vi "SwerveDriveRegisterEachMotor.vi"(8 "error in (no error)":errorcluster, 10 "SwerveDrive refnum name":string="My SwerveDrive RefNum", 11 "SwerveDriveDevRef":T1={"DevStatus"={"status"=FALSE, "code"=0, "source"=""}, "TurnMotors[]"=[], "Square Inputs"=FALSE, "Max Output"=1.0, "DriveMotors[]"=[], "WheelOffset[]"=[], "SwerveSensors[]"=[], "RobotSize"={"Width"=[], "Length"=[], "Center"=[]}}) -> (0 "error out":errorcluster, 3 "SwerveDriveDevRef":T1={"DevStatus"={"status"=FALSE, "code"=0, "source"=""}, "TurnMotors[]"=[], "Square Inputs"=FALSE, "Max Output"=1.0, "DriveMotors[]"=[], "WheelOffset[]"=[], "SwerveSensors[]"=[], "RobotSize"={"Width"=[], "Length"=[], "Center"=[]}})   [LabVIEW 2019, in "Swerve Drive.lvlib"]
doc: "Register each of the motors belonging to RobotDrive."
uses:
  Swerve Drive.lvlib
  SwerveDriveDevRef.ctl
  <vilib>/Rock Robotics/WPI/MotorControl/WPI_MotorControlDeviceRef.ctl
  <vilib>/Rock Robotics/WPI/MotorControl/WPI_MotorControlType.ctl
  <vilib>/Rock Robotics/SystemInterfaces/DIO/FPGA_DIOPWMChannel.ctl
  <vilib>/Rock Robotics/WPI/PWM/WPI_PWMDeadband.ctl
  <vilib>/Rock Robotics/SystemInterfaces/DIO/FPGA_DIOChannel.ctl
  <vilib>/Rock Robotics/SystemInterfaces/AI/FPGA_AIChannel.ctl
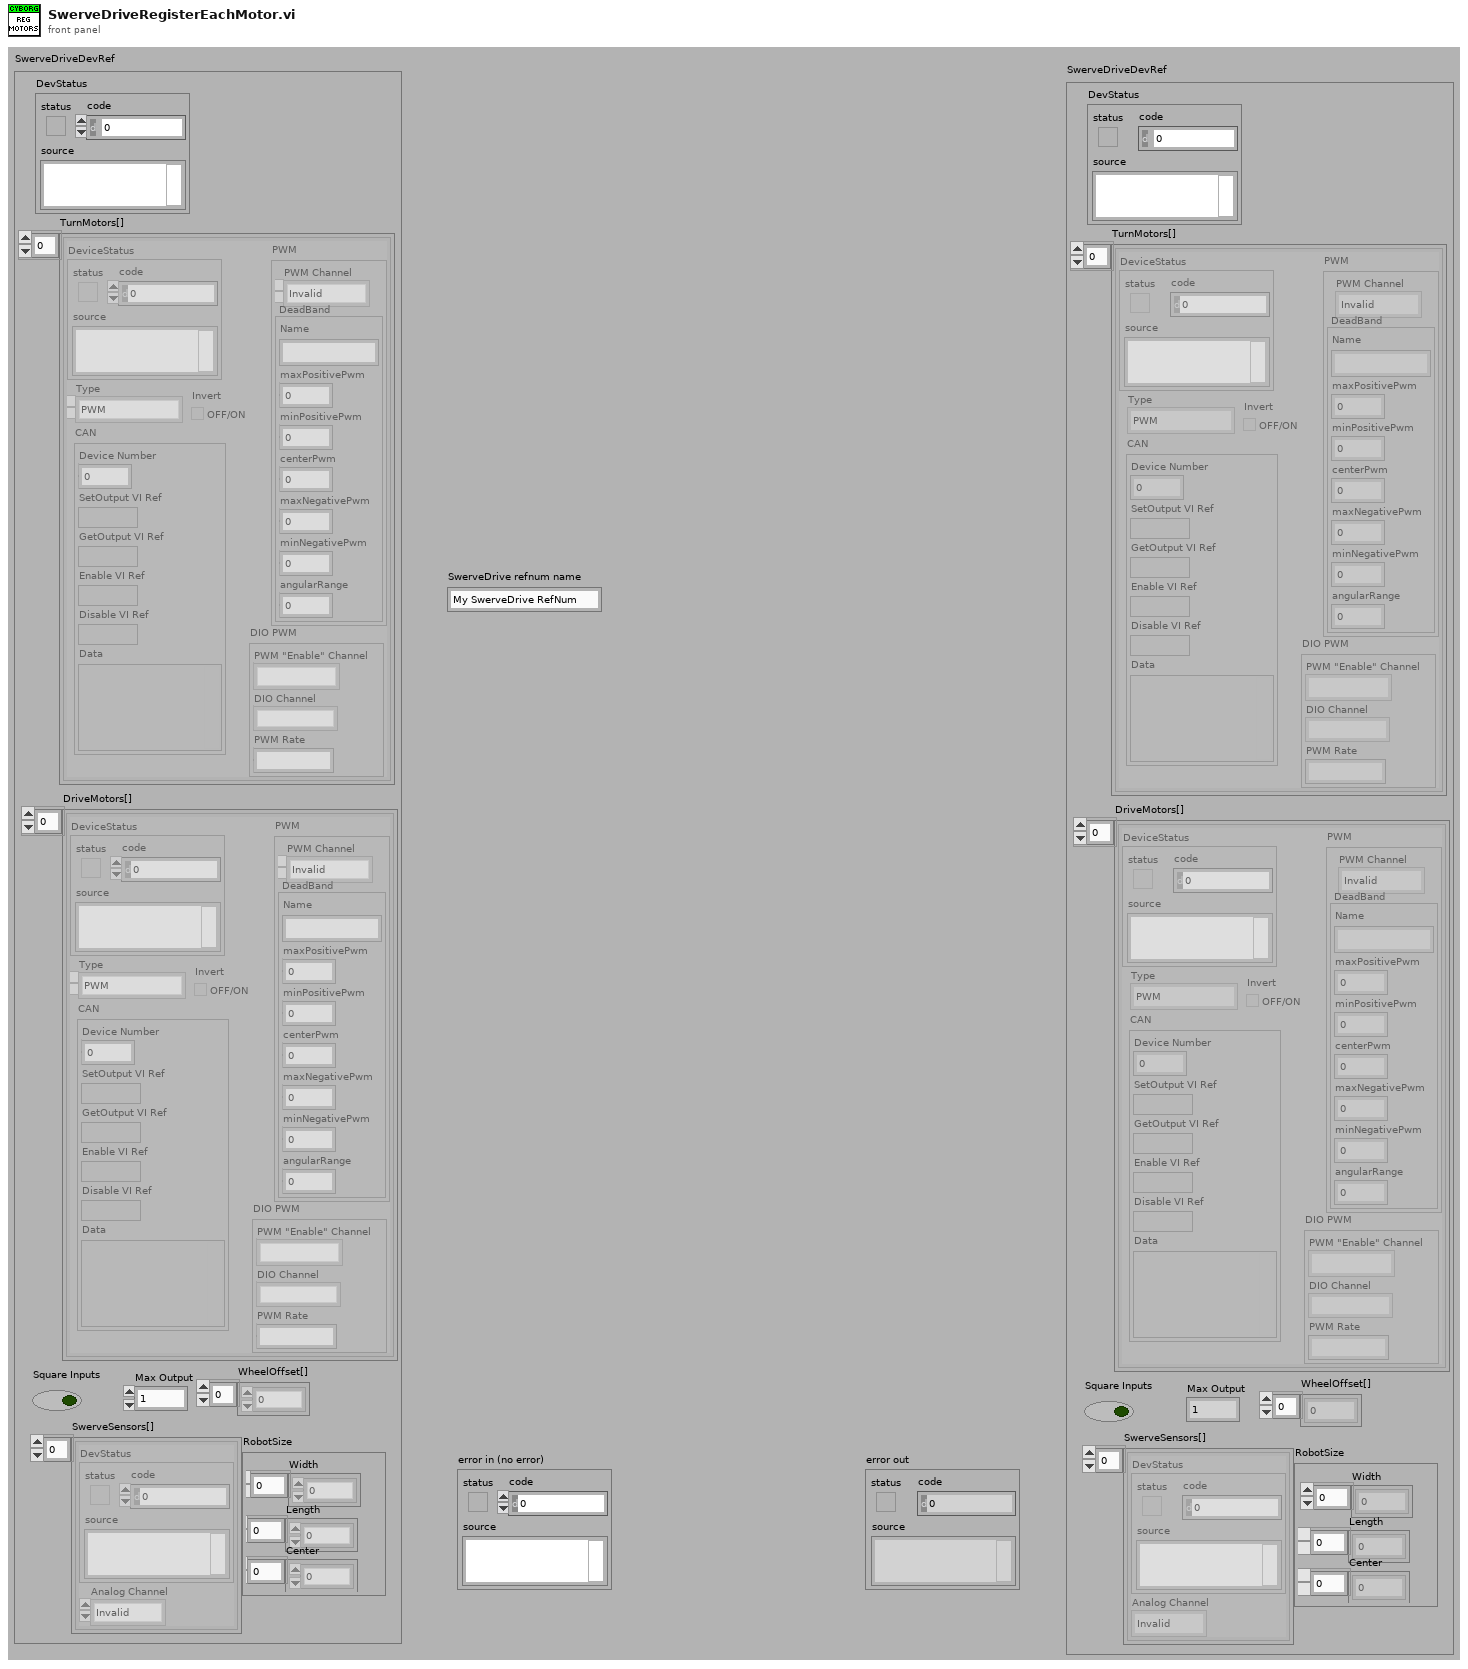
[diagram p1: front panel]
types:
  T1 = typedef "Swerve Drive.lvlib/SwerveDriveDevRef.ctl" = cluster{"DevStatus":errorcluster, "TurnMotors[]":T2[], "Square Inputs":bool, "Max Output":dbl, "DriveMotors[]":T2[], "WheelOffset[]":dbl[], "SwerveSensors[]":cluster{"DevStatus":errorcluster, "Analog Channel":T7}[], "RobotSize":cluster{"Width":dbl[], "Length":dbl[], "Center":dbl[]}}
  T2 = typedef "WPI_MotorControlDeviceRef.ctl" = cluster{"DeviceStatus":errorcluster, "Type":T3, "PWM":cluster{"PWM Channel":T4, "DeadBand":T5}, "CAN":cluster{"Device Number":u8, "SetOutput VI Ref":variant, "GetOutput VI Ref":variant, "Enable VI Ref":variant, "Disable VI Ref":variant, "Data":variant}, "Invert":bool, "DIO PWM":cluster{"PWM \"Enable\" Channel":T4, "DIOChannel":T6, "PWM Rate":dbl}}
  T3 = typedef "WPI_MotorControlType.ctl" = enum16{"PWM", "CAN", "DIO PWM"}
  T4 = typedef "FPGA_DIOPWMChannel.ctl" = enum8{"PWM 0", "PWM 1", "PWM 2", "PWM 3", "PWM 4", "PWM 5", "PWM 6", "PWM 7", "PWM 8", "PWM 9", "PWM MXP 0", "PWM MXP 1", "PWM MXP 2", "PWM MXP 3", "PWM MXP 4", "PWM MXP 5", "PWM MXP 6", "PWM MXP 7", "PWM MXP 8", "PWM MXP 9", "Invalid"}
  T5 = typedef "WPI_PWMDeadband.ctl" = cluster{"Name":string, "maxPositivePwm":i32, "minPositivePwm":i32, "centerPwm":i32, "maxNegativePwm":i32, "minNegativePwm":i32, "angularRange":u16}
  T6 = typedef "FPGA_DIOChannel.ctl" = enum8{"DIO 0", "DIO 1", "DIO 2", "DIO 3", "DIO 4", "DIO 5", "DIO 6", "DIO 7", "DIO 8", "DIO 9", "DIO MXP 0", "DIO MXP 1", "DIO MXP 2", "DIO MXP 3", "DIO MXP 4", "DIO MXP 5", "DIO MXP 6", "DIO MXP 7", "DIO MXP 8", "DIO MXP 9", "DIO MXP 10", "DIO MXP 11", "DIO MXP 12", "DIO MXP 13", "DIO MXP 14", "DIO MXP 15", "SPI Port CS1", "SPI Port CS2", "SPI Port CS3", "SPI Port MISO", "SPI Port MOSI", "Invalid"}
  T7 = typedef "FPGA_AIChannel.ctl" = enum8{"AI 0", "AI 1", "AI 2", "AI 3", "AI MXP 0", "AI MXP 1", "AI MXP 2", "AI MXP 3", "Invalid"}
  T8 = cluster{"DevStatus":errorcluster, "Analog Channel":T7}[]
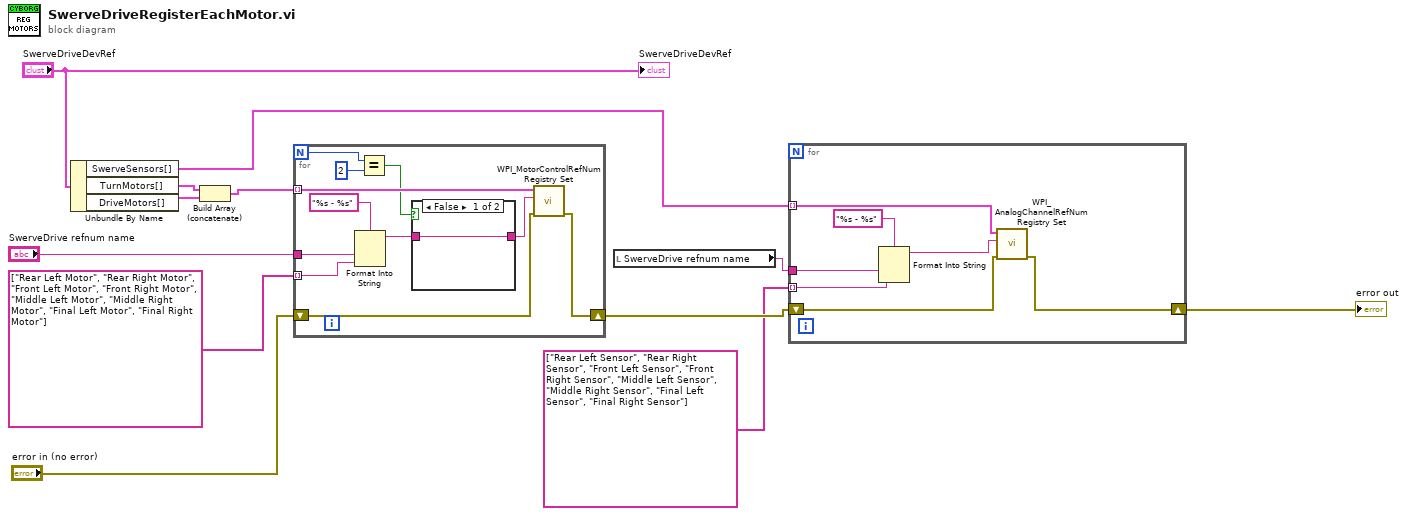
[diagram p0: block diagram]
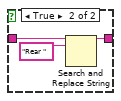
[diagram p2: hidden frame]
diagram:
  n1 = Unbundle By Name("SwerveDriveDevRef") -> ("SwerveSensors[]"=w4:T8, "TurnMotors[]"=w8:T2[], "DriveMotors[]"=w9:T2[])
  n2 = Build Array (concatenate)(w8, w9) -> (w7:T2[])
  n3 = for {
    N -> [w22]
    tunnel: w7 -> [w20] mode=indexing
    tunnel: "SwerveDrive refnum name" -> [w16]
    shift-right: [w14] -> w5
    shift-left: "error in (no error)" -> [w15]
    tunnel: string[] ["Rear Left Motor", "Rear Right Motor", "Front Left Motor", "Front Right Motor", "Middle Left Motor", "Middle Right Motor", "Final Left Motor", "Final Right Motor"] -> [w13] mode=indexing
    n4 = Format Into String(format string="%s - %s", w16, w13) -> (resulting string=w19:string)  [unwired: 2 in, 1 out]
    n5 = Equal?(x=w22, y=2) -> (x = y?=w18:bool)
    n6 = case shown="False" w18 {
      tunnel: w19 -> [w24 w27]
      tunnel: [w24 w26] -> w17
      frame False {
      }
      frame True {
        n7 = Search and Replace String(input string=w27, search string="Rear ") -> (result string=w26:string)  [unwired: 1 in, 8 out]
      }
    }
    n8 = call <vilib>:"WPI_MotorControlRefNum Registry Set.vi"("error in (no error)"=w15, "refnum name"=w17, "MotorControlDevRef"=w20) -> ("error out"=w14:errorcluster)  [unwired: 1 in, 7 out]
  }
  n9 = local read "SwerveDrive refnum name"() -> (w2:string)
  n10 = for {
    shift-right: [w34] -> w6
    shift-left: w5 -> [w33]
    tunnel: w4 -> [w32] mode=indexing
    tunnel: w2 -> [w29]
    tunnel: string[] ["Rear Left Sensor", "Rear Right Sensor", "Front Left Sensor", "Front Right Sensor", "Middle Left Sensor", "Middle Right Sensor", "Final Left Sensor", "Final Right Sensor"] -> [w28] mode=indexing
    n11 = Format Into String(format string="%s - %s", w29, w28) -> (resulting string=w30:string)  [unwired: 2 in, 1 out]
    n12 = call <vilib>:"WPI_AnalogChannelRefNum Registry Set.vi"("error in (no error)"=w33, "refnum name"=w30, "AIDeviceRef"=w32) -> ("error out"=w34:errorcluster)  [unwired: 7 in, 1 out]
  }
  "error out" <- w6
  "SwerveDriveDevRef" <- "SwerveDriveDevRef"
